vi "nigcryo_H_full.vi"() -> ()   [LabVIEW 2019]
uses:
  B_Globals.vi
panel:
  in  "stop":bool
  out "Running Sequence":bool
  out "String":string
  out "Setting Step":dbl=10.348
  out "Field [T]":dbl=10.348
  out "T":cluster{"X":dbl[], "Y":dbl[]}[](graph) caption="XY Graph"
  in  "Go To":bool=TRUE
  in  "Set Field":dbl
  in  "Ramp":bool=TRUE
  in  "Reset Graph":bool
  in  "Rate":dbl=0.2
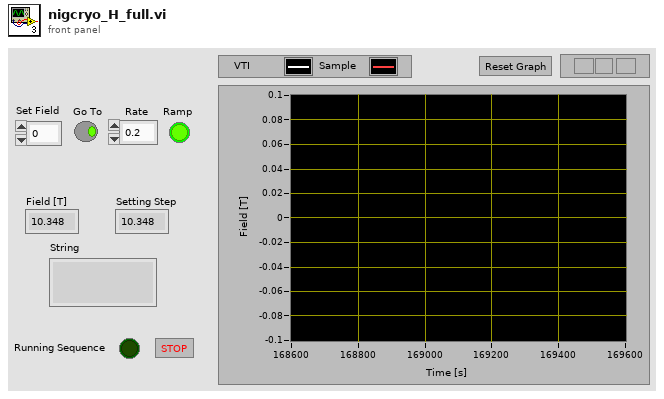
[diagram p1: front panel]
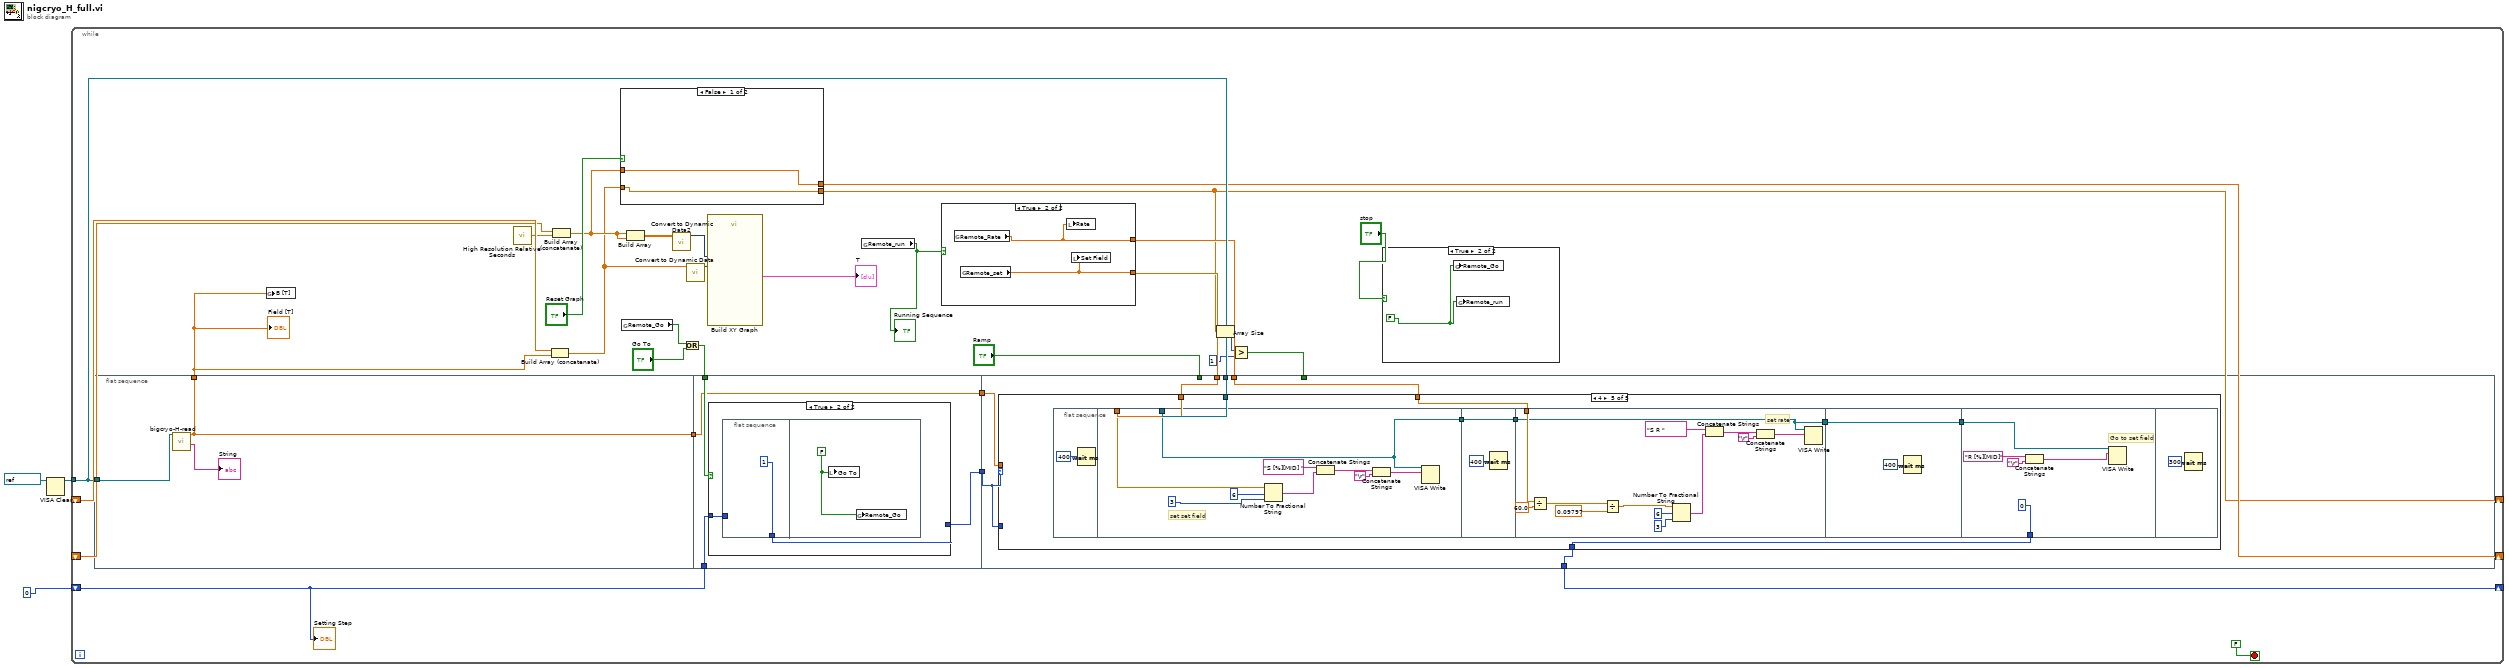
[diagram p0: block diagram]
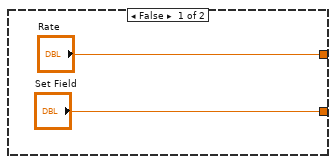
[diagram p3: hidden frame]
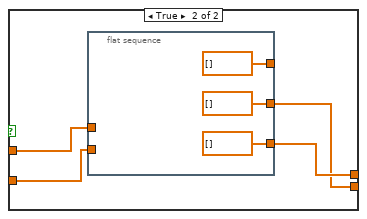
[diagram p4: hidden frame]
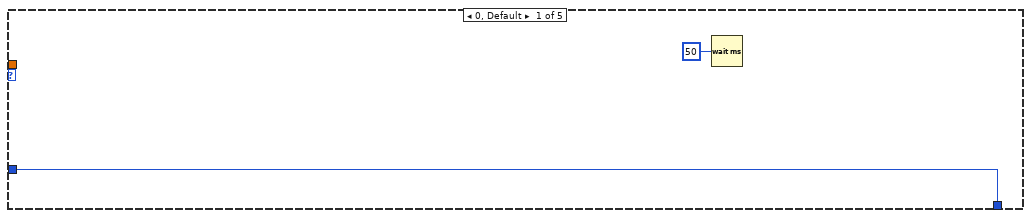
[diagram p6: hidden frame]
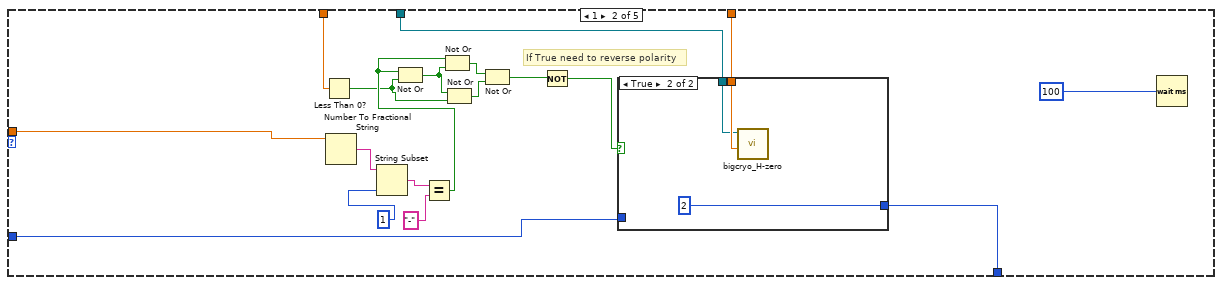
[diagram p7: hidden frame]
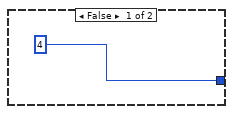
[diagram p8: hidden frame]
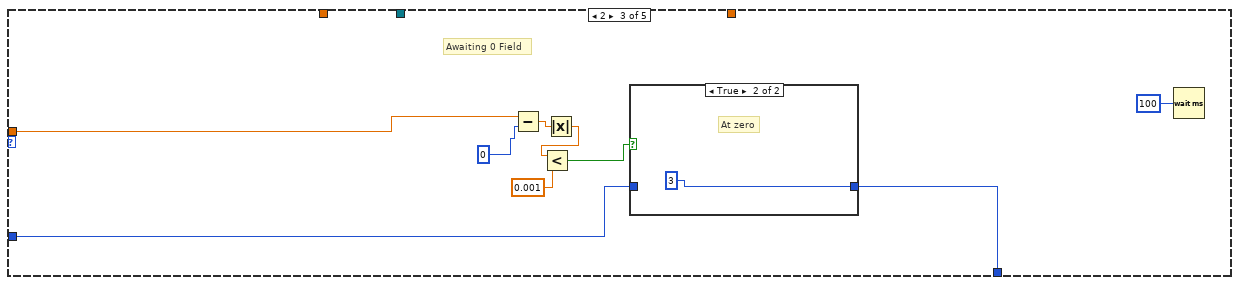
[diagram p9: hidden frame]
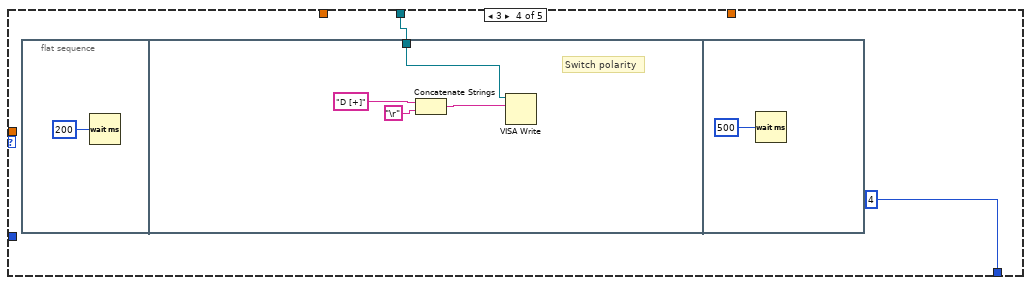
[diagram p11: hidden frame]
diagram:
  n1 = VISA Clear(VISA resource name=refnum<visa-resource-name> "COM6" ("Lakeshore Address")) -> (VISA resource name out=w3:refnum<visa-resource-name>)  [unwired: 1 in, 1 out]
  n2 = while {
    tunnel: w3 -> [w25]
    shift-right: [w19] -> _
    shift-left: _ -> [w33]
    shift-right: [w21] -> _
    shift-left: _ -> [w31]
    shift-right: [w10] -> _
    shift-left: 0 -> [w9]
    stop <- FALSE stop-if-true
    n3 = flat-sequence {
      tunnel: [w51] -> w13
      tunnel: [w51] -> w14
      tunnel: w25 -> [w50]
      tunnel: w6 -> [w55]
      tunnel: w13 -> [w52]
      tunnel: w9 -> [w54]
      tunnel: [w53] -> w12
      tunnel: [w52] -> w11
      tunnel: [w63] -> w10
      tunnel: w11 -> [w66]
      tunnel: w12 -> [w64]
      tunnel: w17 -> [_]
      tunnel: w22 -> [w62]
      tunnel: "Ramp" -> [_]
      tunnel: w24 -> [w65]
      tunnel: w25 -> [w61]
      frame #0 {
        n4 = call "bigcryo-H-read.vi"("Magnet Power supply"=w50) -> ("substring"=→"String":string, "Magnetic Field [T]"=w51:dbl)  [unwired: 9 in]
      }
      frame #1 {
        n5 = case shown="True" w55 {
          tunnel: w54 -> [w56 w58]
          tunnel: [w56 w57] -> w53
          frame False {
          }
          frame True {
            n6 = flat-sequence {
              tunnel: w58 -> [_]
              tunnel: [1] -> w57
              frame #0 {
              }
              frame #1 {
                w60 = FALSE
                n7 = local write "Go To"(w60) -> ()
                n8 = global write "B_Globals.vi" "Remote_Go"(w60) -> ()
              }
            }
          }
        }
      }
      frame #2 {
        n9 = case shown="4" w64 {
          tunnel: w66 -> [_ w82 w96 _ _]
          tunnel: w65 -> [_ w77 _ _ w116]
          tunnel: w64 -> [w68 w74 w93 _ _]
          tunnel: [w68 w73 w92 4 w110] -> w63
          tunnel: w62 -> [_ w71 _ _ w113]
          tunnel: w61 -> [_ w70 _ w103 w117]
          frame 0, Default {
            n10 = Wait (ms)(milliseconds to wait=50) -> ()  [unwired: 1 out]
          }
          frame 1 {
            # "If True need to reverse polarity"
            n11 = Less Than 0?(x=w77) -> (x < 0?=w72:bool)
            n12 = Number To Fractional String(number=w82) -> (F-format string=w85:string)  [unwired: 3 in]
            n13 = String Subset(string=w85, length (rest)=1 ("length (rest)")) -> (substring=w84:string)  [unwired: 1 in]
            n14 = Equal?(x=w84, y="-") -> (x = y?=w76:bool)
            n15 = Not Or(1:w72, 2:w76) -> (0:w81:bool)
            n16 = Not Or(1:w81, 2:w76) -> (0:w80:bool)
            n17 = Not Or(1:w72, 2:w81) -> (0:w79:bool)
            n18 = Not Or(1:w79, 2:w80) -> (0:w78:bool)
            n19 = Not(x=w78) -> (.not. x?=w75:bool)
            n20 = case shown="True" w75 {
              tunnel: w74 -> [_ _]
              tunnel: [4 2] -> w73
              tunnel: w71 -> [_ w89]
              tunnel: w70 -> [_ w88]
              frame False {
              }
              frame True {
                n21 = call "bigcryo_H-zero.vi"("Rate [T/min]"=w89, "Magnet Power supply"=w88) -> ()  [unwired: 10 in]
              }
            }
            n22 = Wait (ms)(milliseconds to wait=100) -> ()  [unwired: 1 out]
          }
          frame 2 {
            # "Awaiting 0 Field"
            n23 = Subtract(x=w96, y=0) -> (x-y=w98:dbl)
            n24 = Absolute Value(x=w98) -> (abs(x)=w95:dbl)
            n25 = Less?(x=w95, y=0.001) -> (x < y?=w94:bool)
            n26 = case shown="True" w94 {
              tunnel: w93 -> [w100 _]
              tunnel: [w100 3] -> w92
              frame False {
              }
              frame True {
                # "At zero"
              }
            }
            n27 = Wait (ms)(milliseconds to wait=100) -> ()  [unwired: 1 out]
          }
          frame 3 {
            n28 = flat-sequence {
              tunnel: w103 -> [w105]
              frame #0 {
                n29 = Wait (ms)(milliseconds to wait=200) -> ()  [unwired: 1 out]
              }
              frame #1 {
                # "Switch polarity"
                n30 = Concatenate Strings("D [+]" ("data"), "\r") -> (w108:string)
                n31 = VISA Write(VISA resource name=w105, write buffer=w108) -> ()  [unwired: 1 in, 3 out]
              }
              frame #2 {
                n32 = Wait (ms)(milliseconds to wait=500) -> ()  [unwired: 1 out]
              }
            }
          }
          frame 4 {
            n33 = flat-sequence {
              tunnel: w117 -> [w119]
              tunnel: w116 -> [w120]
              tunnel: [w119] -> w114
              tunnel: [w128] -> w115
              tunnel: w114 -> [w128]
              tunnel: w115 -> [w130]
              tunnel: w113 -> [w131]
              tunnel: [w130] -> w111
              tunnel: [w144] -> w112
              tunnel: w111 -> [w144]
              tunnel: w112 -> [w146]
              tunnel: [0] -> w110
              frame #0 {
                n34 = Wait (ms)(milliseconds to wait=400) -> ()  [unwired: 1 out]
              }
              frame #1 {
                # "set set field"
                n35 = Number To Fractional String(number=w120, width (-)=i16 6, precision (6)=i16 3) -> (F-format string=w124:string)  [unwired: 1 in]
                n36 = Concatenate Strings("S [%][MID] " ("string"), w124) -> (w121:string)
                n37 = Concatenate Strings(w121, "\r") -> (w123:string)
                n38 = VISA Write(VISA resource name=w119, write buffer=w123) -> ()  [unwired: 1 in, 3 out]
              }
              frame #2 {
                n39 = Wait (ms)(milliseconds to wait=400) -> ()  [unwired: 1 out]
              }
              frame #3 {
                # "set rate"
                n40 = Divide(x=w131, y=60.0) -> (x/y=w136:dbl)
                n41 = Divide(x=w136, y=0.09797) -> (x/y=w134:dbl)
                n42 = Number To Fractional String(number=w134, width (-)=i16 6, precision (6)=i16 3) -> (F-format string=w139:string)  [unwired: 1 in]
                n43 = Concatenate Strings("S R " ("string"), w139) -> (w138:string)
                n44 = Concatenate Strings(w138, "\r") -> (w142:string)
                n45 = VISA Write(VISA resource name=w130, write buffer=w142) -> ()  [unwired: 1 in, 3 out]
              }
              frame #4 {
                n46 = Wait (ms)(milliseconds to wait=400) -> ()  [unwired: 1 out]
              }
              frame #5 {
                # "Go to set field"
                n47 = Concatenate Strings("R [%][MID]" ("data"), "\r") -> (w149:string)
                n48 = VISA Write(VISA resource name=w146, write buffer=w149) -> ()  [unwired: 1 in, 3 out]
              }
              frame #6 {
                n49 = Wait (ms)(milliseconds to wait=300) -> ()  [unwired: 1 out]
              }
            }
          }
        }
      }
    }
    n50 = global write "B_Globals.vi" "B [T]"(w14) -> ()
    n51 = call <vilib>:"High Resolution Relative Seconds.vi"() -> ("relative seconds"=w30:dbl)
    n52 = Build Array (concatenate)(w33, w14) -> (w16:dbl[])
    n53 = Build Array (concatenate)(w31, w30) -> (w26:dbl[])
    n54 = case shown="False" "Reset Graph" {
      tunnel: w26 -> [w41 w45]
      tunnel: [w41 w44] -> w21
      tunnel: [w40 w43] -> w19
      tunnel: w16 -> [w40 w42]
      frame False {
      }
      frame True {
        n55 = flat-sequence {
          tunnel: w45 -> [_]
          tunnel: [dbl[] []] -> _
          tunnel: [dbl[] []] -> w44
          tunnel: [dbl[] []] -> w43
          tunnel: w42 -> [_]
          frame #0 {
          }
        }
      }
    }
    n56 = global read "B_Globals.vi" "Remote_Go"() -> (w8:bool)
    n57 = Build Array(w26, w26) -> (w29:dbl[][])
    n58 = call "Convert to Dynamic Data2"("2D Array"=w29) -> ("Dynamic Data Type"=w28:dynamicdata)  [unwired: 3 in]
    n59 = Or(x=w8, y="Go To") -> (x .or. y?=w6:bool)
    n60 = call "Convert to Dynamic Data"("Array"=w16) -> ("Dynamic Data Type"=w15:dynamicdata)  [unwired: 3 in]
    n61 = call "Build XY Graph"("Y Input"=w15, "X Input"=w28) -> ("XY Graph"=→"T":cluster{"X":dbl[], "Y":dbl[]}[])  [unwired: 8 in, 1 out]
    n62 = global read "B_Globals.vi" "Remote_run"() -> (w5:bool)
    "Running Sequence" <- w5
    n63 = case shown="True" w5 {
      tunnel: ["Set Field" w38] -> w24
      tunnel: ["Rate" w39] -> w22
      frame False {
      }
      frame True {
        n64 = global read "B_Globals.vi" "Remote_Rate"() -> (w39:dbl)
        n65 = global read "B_Globals.vi" "Remote_set"() -> (w38:dbl)
        n66 = local write "Rate"(w39) -> ()
        n67 = local write "Set Field"(w38) -> ()
      }
    }
    n68 = Array Size(array=w19) -> (size(s)=w20:i32)
    n69 = Greater?(x=w20, y=1) -> (0:w17:bool)
    n70 = case shown="True" "stop" {
      frame False {
      }
      frame True {
        w35 = FALSE
        n71 = global write "B_Globals.vi" "Remote_Go"(w35) -> ()
        n72 = global write "B_Globals.vi" "Remote_run"(w35) -> ()
      }
    }
    "Field [T]" <- w14
    "Setting Step" <- w9
  }
